vi "Slack-Sign In With Slack.vi"(0 "client_id":string="1023330033985.1023512746241", 5 "client_secret":string="62f876b60829c507c6cb25bfe9dbba2b") -> (4 "user":T1, 15 "error out":errorcluster)   [LabVIEW 2015]
uses:
  Slack-User.ctl
  <vilib>/Platform/browser.llb/Open URL in Default Browser (string).vi
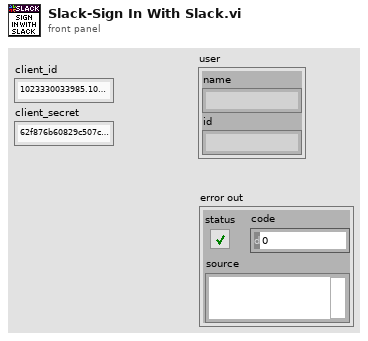
[diagram p1: front panel]
types:
  T1 = typedef "Slack-User.ctl" = cluster{"name":string, "id":string}
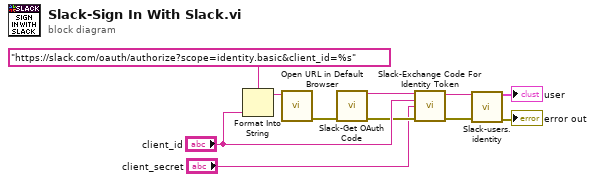
[diagram p0: block diagram]
diagram:
  n1 = Format Into String(format string="https://slack.com/oauth/authorize?scope=identity.basic&client_id=%s", "client_id") -> (resulting string=w9:string)  [unwired: 2 in, 1 out]
  n2 = call-poly <vilib>:"Open URL in Default Browser.vi"("URL"=w9) -> ("error out"=w5:errorcluster)  [unwired: 5 in, 1 out]
  n3 = call "Slack-Get OAuth Code.vi"("error in (no error)"=w5) -> ("code"=w6:string, "error out"=w8:errorcluster)  [unwired: 13 in]
  n4 = call "Slack-Exchange Code For Identity Token.vi"("code"=w6, "client_id"="client_id", "client_secret"="client_secret", "error in (no error)"=w8) -> ("access_token"=w4:string, "error out"=w3:errorcluster)  [unwired: 10 in]
  n5 = call "Slack-users.identity.vi"("token"=w4, "error in (no error)"=w3) -> ("user"=→"user":T1, "error out"=→"error out":errorcluster)  [unwired: 12 in]
